vi "LED Controls.vi"(2 "Enum":enum16{"Start", "Run", "End"}(ring)) -> ()   [LabVIEW 2013]
uses:
  Team Code/Robot Global Data.vi
  <vilib>/Rock Robotics/SystemInterfaces/DIO/FPGA_DIOChannel.ctl
  <vilib>/Rock Robotics/SystemInterfaces/Typedef/FPGA_TypedefDigitalModule.ctl
  TypeDefs/Digital Module 1.ctl
panel:
  in  "LED state":dbl
  in  "Digital Module A":T1={"Module"=enum."Digital Module 1", "L Encoder A"=enum."DIO 1", "L Encoder B"=enum."DIO 2", "R Encoder A"=enum."DIO 3", "R Encoder B"=enum."DIO 4", "Compressor"=enum."DIO 5", "Shooter Limit"=enum."DIO 6", "LED 1"=enum."DIO 7", "LED 2"=enum."DIO 8", "LED 3"=enum."DIO 9", "LED 4"=enum."DIO 10", "Shooter Limit 2"=enum."DIO 11", "Unassigned"=enum."DIO 12", "Unassigned"=enum."DIO 13", "Unassigned"=enum."DIO 14"}
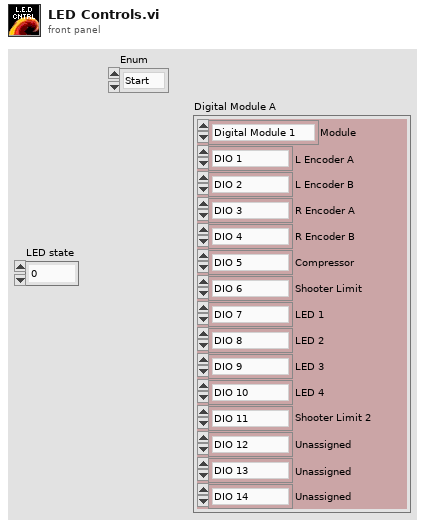
[diagram p1: front panel]
types:
  T1 = typedef "Digital Module 1.ctl" = cluster{"Module":T2, "L Encoder A":T3, "L Encoder B":T3, "R Encoder A":T3, "R Encoder B":T3, "Compressor":T3, "Shooter Limit":T3, "LED 1":T3, "LED 2":T3, "LED 3":T3, "LED 4":T3, "Shooter Limit 2":T3, "Unassigned":T3, "Unassigned":T3, "Unassigned":T3}
  T2 = typedef "FPGA_TypedefDigitalModule.ctl" = enum16{"Digital Module 1", "Digital Module 2"}
  T3 = typedef "FPGA_DIOChannel.ctl" = enum8{"DIO 1", "DIO 2", "DIO 3", "DIO 4", "DIO 5", "DIO 6", "DIO 7", "DIO 8", "DIO 9", "DIO 10", "DIO 11", "DIO 12", "DIO 13", "DIO 14", "Invalid"}
  T4 = enum16{"Nothing", "Load", "Lock", "Pass", "Grab", "Loader Down", "Shoot", "Auto Start", "Tele Start"}
  T5 = typedef "WPI_DigitalOutputDevRef.ctl" = cluster{"Digital Module":T2, "DIO Channel":T3, "DevStatus":errorcluster}
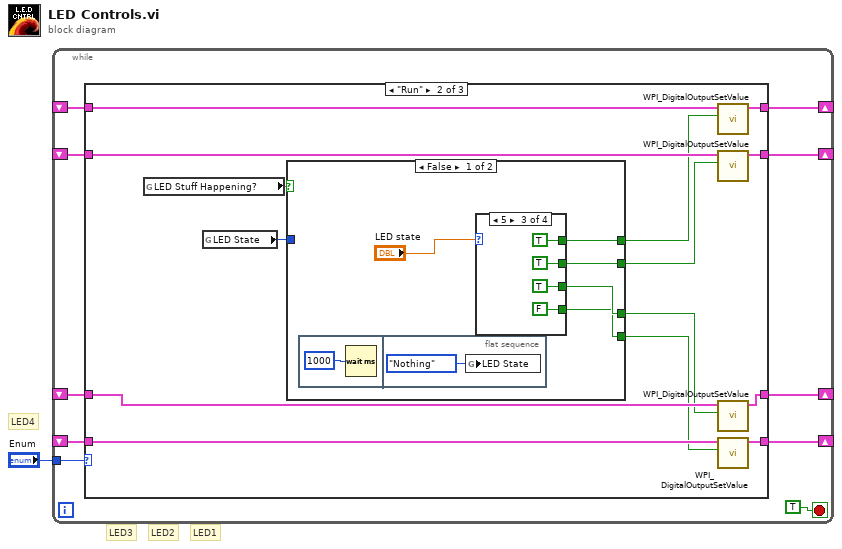
[diagram p0: block diagram]
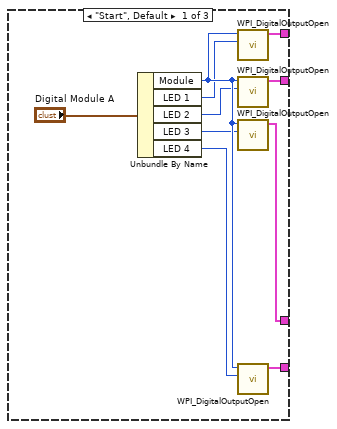
[diagram p2: hidden frame]
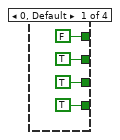
[diagram p3: hidden frame]
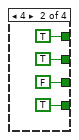
[diagram p4: hidden frame]
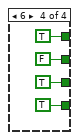
[diagram p5: hidden frame]
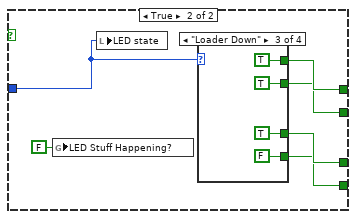
[diagram p6: hidden frame]
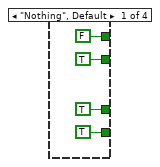
[diagram p7: hidden frame]
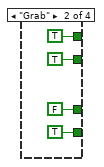
[diagram p8: hidden frame]
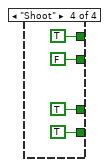
[diagram p9: hidden frame]
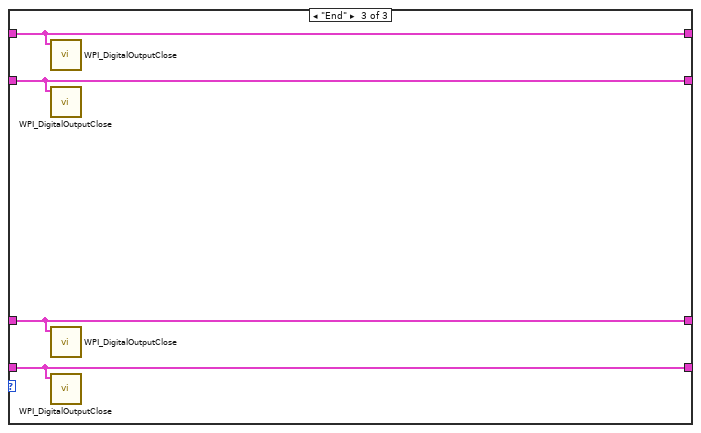
[diagram p10: hidden frame]
diagram:
  # "LED4"
  # "LED3"
  # "LED2"
  # "LED1"
  n1 = while {
    tunnel: "Enum" -> [w10]
    shift-right: [w8] -> _
    shift-left: _ -> [w9]
    shift-right: [w7] -> _
    shift-left: _ -> [w4]
    shift-right: [w6] -> _
    shift-left: _ -> [w3]
    shift-right: [w5] -> _
    shift-left: _ -> [w2]
    stop <- TRUE stop-if-true
    n2 = case shown="\"Run\"" w10 {
      tunnel: w9 -> [_ w31 w81]
      tunnel: [w20 w35 w81] -> w8
      tunnel: [w19 w34 w82] -> w7
      tunnel: [w18 w33 w83] -> w6
      tunnel: [w17 w32 w84] -> w5
      tunnel: w4 -> [_ w30 w82]
      tunnel: w3 -> [_ w29 w83]
      tunnel: w2 -> [_ w28 w84]
      frame "Start", Default {
        n3 = Unbundle By Name("Digital Module A") -> ("Module"=w16:T2, "LED 1"=w12:T3, "LED 2"=w13:T3, "LED 3"=w14:T3, "LED 4"=w15:T3)
        n4 = call <vilib>:"WPI_DigitalOutputOpen.vi"("DIO Channel"=w12, "Digital Module (Module 1)"=w16) -> ("DigitalOutputDevRef"=w20:T5)  [unwired: 8 in, 1 out]
        n5 = call <vilib>:"WPI_DigitalOutputOpen.vi"("DIO Channel"=w13, "Digital Module (Module 1)"=w16) -> ("DigitalOutputDevRef"=w19:T5)  [unwired: 8 in, 1 out]
        n6 = call <vilib>:"WPI_DigitalOutputOpen.vi"("DIO Channel"=w14, "Digital Module (Module 1)"=w16) -> ("DigitalOutputDevRef"=w18:T5)  [unwired: 8 in, 1 out]
        n7 = call <vilib>:"WPI_DigitalOutputOpen.vi"("DIO Channel"=w15, "Digital Module (Module 1)"=w16) -> ("DigitalOutputDevRef"=w17:T5)  [unwired: 8 in, 1 out]
      }
      frame "Run" {
        n8 = global read "Robot Global Data.vi" "LED Stuff Happening?"() -> (w22)
        n9 = global read "Robot Global Data.vi" "LED State"() -> (w23:T4)
        n10 = case shown="False" w22 {
          tunnel: [w40 w64] -> w27
          tunnel: [w39 w63] -> w26
          tunnel: [w38 w62] -> w25
          tunnel: [w37 w61] -> w24
          tunnel: w23 -> [_ w60]
          frame False {
            n11 = flat-sequence {
              frame #0 {
                n12 = Wait (ms)(milliseconds to wait=u32 1000) -> ()  [unwired: 1 out]
              }
              frame #1 {
                n13 = global write "Robot Global Data.vi" "LED State"(T4."Nothing" ("LED State")) -> ()
              }
            }
            n14 = case shown="5" "LED state" {
              tunnel: [FALSE TRUE TRUE TRUE] -> w40
              tunnel: [TRUE TRUE TRUE FALSE] -> w39
              tunnel: [TRUE FALSE TRUE TRUE] -> w38
              tunnel: [TRUE TRUE FALSE TRUE] -> w37
              frame 0, Default {
              }
              frame 4 {
              }
              frame 5 {
              }
              frame 6 {
              }
            }
          }
          frame True {
            n15 = global write "Robot Global Data.vi" "LED Stuff Happening?"(FALSE ("LED Stuff Happening?")) -> ()
            n16 = local write "LED state"(w60) -> ()
            n17 = case shown="\"Loader Down\"" w60 {
              tunnel: [FALSE TRUE TRUE TRUE] -> w64
              tunnel: [TRUE TRUE TRUE FALSE] -> w63
              tunnel: [TRUE FALSE TRUE TRUE] -> w62
              tunnel: [TRUE TRUE FALSE TRUE] -> w61
              frame "Nothing", Default {
              }
              frame "Grab" {
              }
              frame "Loader Down" {
              }
              frame "Shoot" {
              }
            }
          }
        }
        n18 = call <vilib>:"WPI_DigitalOutputSetValue.vi"("Value"=w27, "DigitalOutputDevRef"=w31) -> ("DigitalOutputDevRef"=w35:T5)  [unwired: 8 in, 1 out]
        n19 = call <vilib>:"WPI_DigitalOutputSetValue.vi"("Value"=w26, "DigitalOutputDevRef"=w30) -> ("DigitalOutputDevRef"=w34:T5)  [unwired: 8 in, 1 out]
        n20 = call <vilib>:"WPI_DigitalOutputSetValue.vi"("Value"=w25, "DigitalOutputDevRef"=w29) -> ("DigitalOutputDevRef"=w33:T5)  [unwired: 8 in, 1 out]
        n21 = call <vilib>:"WPI_DigitalOutputSetValue.vi"("Value"=w24, "DigitalOutputDevRef"=w28) -> ("DigitalOutputDevRef"=w32:T5)  [unwired: 8 in, 1 out]
      }
      frame "End" {
        n22 = call <vilib>:"WPI_DigitalOutputClose.vi"("DigitalOutputDevRef"=w81) -> ()  [unwired: 10 in, 1 out]
        n23 = call <vilib>:"WPI_DigitalOutputClose.vi"("DigitalOutputDevRef"=w82) -> ()  [unwired: 10 in, 1 out]
        n24 = call <vilib>:"WPI_DigitalOutputClose.vi"("DigitalOutputDevRef"=w83) -> ()  [unwired: 10 in, 1 out]
        n25 = call <vilib>:"WPI_DigitalOutputClose.vi"("DigitalOutputDevRef"=w84) -> ()  [unwired: 10 in, 1 out]
      }
    }
  }
